vi "dfd_Classical FIR Order Checker.vi"(7 "filter type":T1(ring), 8 "error in (no error)":errorcluster, 10 "order option":enum16{"MinNum", "MinEven", "MinOdd"}(ring), 11 "order in":i32) -> (0 "error out":errorcluster, 3 "order out":i32)   [LabVIEW 2017, in "NI_DigFilterLicensed.lvlib"]
uses:
  <vilib>/addons/Digital Filter Design/NI_DigFilterLicensed.lvlib
  <vilib>/addons/Digital Filter Design/_Misc.llb/dfd_Error Cluster From Error Code (Scalar).vi
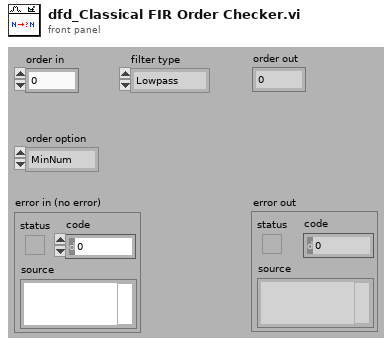
[diagram p1: front panel]
types:
  T1 = enum16{"Lowpass", "Highpass", "Bandpass", "Bandstop"}
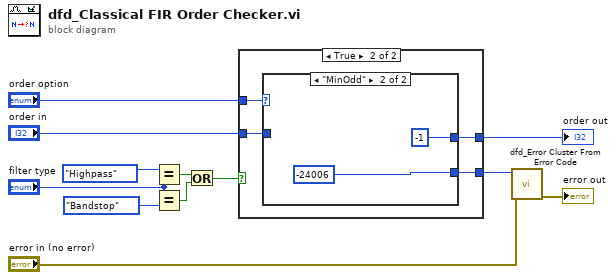
[diagram p0: block diagram]
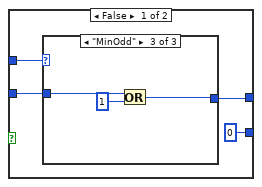
[diagram p2: hidden frame]
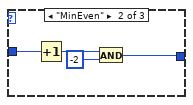
[diagram p4: hidden frame]
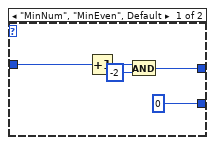
[diagram p5: hidden frame]
diagram:
  n1 = Equal?(x=T1."Highpass" ("filter type"), y="filter type") -> (x = y?=w7:bool)
  n2 = Equal?(x="filter type", y=T1."Bandstop" ("filter type")) -> (x = y?=w6:bool)
  n3 = Or(x=w7, y=w6) -> (x .or. y?=w9:bool)
  n4 = case shown="True" w9 {
    tunnel: "order in" -> [w15 w27]
    tunnel: "order option" -> [w16 w28]
    tunnel: [w14 w26] -> w12
    tunnel: [0 w25] -> w3
    frame False {
      n5 = case shown="\"MinOdd\"" w16 {
        tunnel: w15 -> [w17 w21 w24]
        tunnel: [w17 w18 w22] -> w14
        frame "MinNum", Default {
        }
        frame "MinEven" {
          n6 = Increment(x=w21) -> (x+1=w20:i32)
          n7 = And(x=w20, y=-2) -> (x .and. y?=w18:i32)
        }
        frame "MinOdd" {
          n8 = Or(x=w24, y=1) -> (x .or. y?=w22:i32)
        }
      }
    }
    frame True {
      n9 = case shown="\"MinOdd\"" w28 {
        tunnel: w27 -> [w33 _]
        tunnel: [w30 -1] -> w26
        tunnel: [0 -24006 ("ERR_TYPE_II_HIGHPASS")] -> w25
        frame "MinNum", "MinEven", Default {
          n10 = Increment(x=w33) -> (x+1=w32:i32)
          n11 = And(x=w32, y=-2) -> (x .and. y?=w30:i32)
        }
        frame "MinOdd" {
        }
      }
    }
  }
  "order out" <- w12
  n12 = call-poly <vilib>:"dfd_Error Cluster From Error Code.vi"("error in (no error)"="error in (no error)", "error code (0)"=w3) -> ("error out"=→"error out":errorcluster)  [unwired: 9 out]
